vi "A3-GPS-Decoder.vi"(2 "ASCII Hexidecimal String":string) -> (0 "Date (YYYYMMDD)":u32, 1 "Time (HHMMSS)":u32, 3 "Longitude (Deg)":dbl, 4 "Latitude (Deg)":dbl, 5 "AMSL (m)":sgl, 6 "Velocity North (cm/s)":sgl, 7 "Velocity East (cm/s)":sgl, 8 "Velocity Down (cm/s)":sgl)   [LabVIEW 2019]
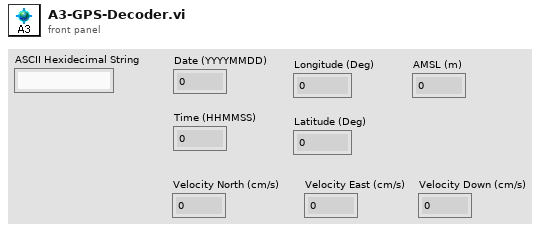
[diagram p1: front panel]
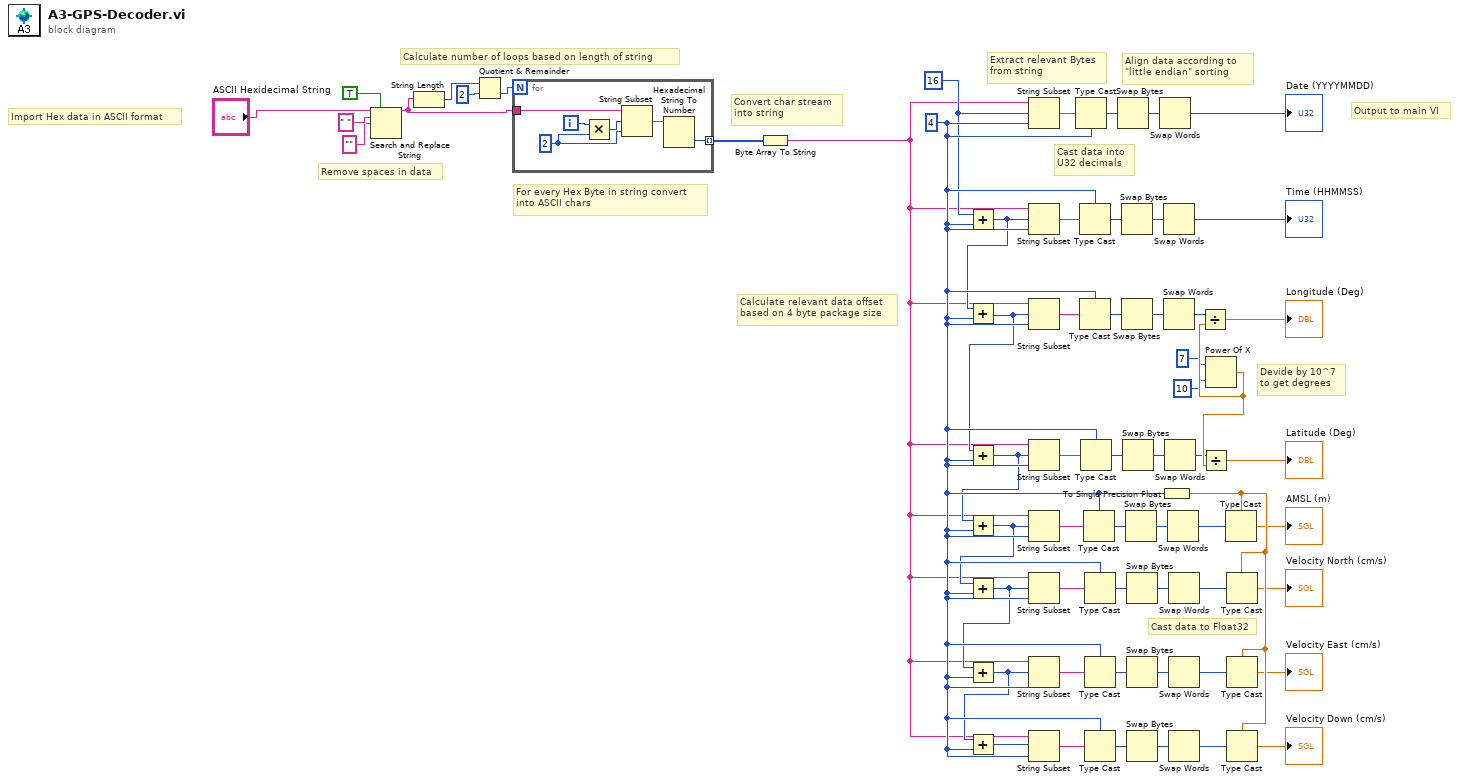
[diagram p0: block diagram]
diagram:
  w61 = u32 4 ("length (rest)")
  w20 = u32 16 ("offset (0)")
  # "Calculate relevant data offset \nbased on 4 byte package size"
  # "Cast data to Float32"
  # "Devide by 10^7 \nto get degrees"
  # "Output to main VI"
  # "Align data according to \n\"little endian\" sorting"
  # "Cast data into \nU32 decimals"
  # "Extract relevant Bytes \nfrom string"
  # "Convert char stream\ninto string"
  # "For every Hex Byte in string convert \ninto ASCII chars"
  # "Calculate number of loops based on length of string"
  # "Remove spaces in data"
  # "Import Hex data in ASCII format"
  n1 = Search and Replace String(replace all?=TRUE ("replace all? (F)"), input string="ASCII Hexidecimal String", search string=" ", replace string="" ("replace string (\"\")")) -> (result string=w3:string)  [unwired: 4 in, 3 out]
  n2 = String Length(string=w3) -> (length=w10:i32)
  n3 = Quotient & Remainder(x=w10, y=2) -> (floor(x/y)=w8:i32)  [unwired: 1 out]
  n4 = for {
    N: w8 -> [_]
    tunnel: w3 -> [w62]
    tunnel: [w63] -> w7 mode=indexing
    i -> [w66]
    w65 = 2 ("length (rest)")
    n5 = Multiply(x=w66, y=w65) -> (x*y=w67:i32)
    n6 = String Subset(string=w62, offset (0)=w67, length (rest)=w65) -> (substring=w64:string)
    n7 = Hexadecimal String To Number(string=w64) -> (number=w63:u32)  [unwired: 2 in, 1 out]
  }
  n8 = Byte Array To String(unsigned byte array=w7) -> (string=w2:string)
  n9 = Add(x=w20, y=w61) -> (x+y=w21:u32)
  n10 = Add(x=w21, y=w61) -> (x+y=w30:u32)
  n11 = Add(x=w30, y=w61) -> (x+y=w33:u32)
  n12 = Add(x=w33, y=w61) -> (x+y=w41:u32)
  n13 = Add(x=w41, y=w61) -> (x+y=w60:u32)
  n14 = Add(x=w60, y=w61) -> (x+y=w50:u32)
  n15 = Add(x=w50, y=w61) -> (x+y=w58:u32)
  n16 = String Subset(string=w2, offset (0)=w20, length (rest)=w61) -> (substring=w11:string)
  n17 = String Subset(string=w2, offset (0)=w21, length (rest)=w61) -> (substring=w51:string)
  n18 = String Subset(string=w2, offset (0)=w30, length (rest)=w61) -> (substring=w52:string)
  n19 = String Subset(string=w2, offset (0)=w33, length (rest)=w61) -> (substring=w53:string)
  n20 = String Subset(string=w2, offset (0)=w41, length (rest)=w61) -> (substring=w54:string)
  n21 = String Subset(string=w2, offset (0)=w60, length (rest)=w61) -> (substring=w55:string)
  n22 = String Subset(string=w2, offset (0)=w50, length (rest)=w61) -> (substring=w56:string)
  n23 = String Subset(string=w2, offset (0)=w58, length (rest)=w61) -> (substring=w57:string)
  n24 = Type Cast(type=w61, x=w11) -> (*(type *) &x=w13:u32)
  n25 = Type Cast(type=w61, x=w51) -> (*(type *) &x=w16:u32)
  n26 = Type Cast(type=w61, x=w52) -> (*(type *) &x=w19:u32)
  n27 = Type Cast(type=w61, x=w53) -> (*(type *) &x=w27:u32)
  n28 = Type Cast(type=w61, x=w54) -> (*(type *) &x=w34:u32)
  n29 = Type Cast(type=w61, x=w55) -> (*(type *) &x=w38:u32)
  n30 = Type Cast(type=w61, x=w56) -> (*(type *) &x=w43:u32)
  n31 = Type Cast(type=w61, x=w57) -> (*(type *) &x=w47:u32)
  n32 = Swap Bytes(anything=w13) -> (byte swapped=w12:u32)
  n33 = Swap Bytes(anything=w16) -> (byte swapped=w15:u32)
  n34 = Swap Bytes(anything=w19) -> (byte swapped=w18:u32)
  n35 = Swap Bytes(anything=w27) -> (byte swapped=w26:u32)
  n36 = Swap Bytes(anything=w34) -> (byte swapped=w32:u32)
  n37 = Swap Bytes(anything=w38) -> (byte swapped=w37:u32)
  n38 = Swap Bytes(anything=w43) -> (byte swapped=w42:u32)
  n39 = Swap Bytes(anything=w47) -> (byte swapped=w46:u32)
  n40 = Swap Words(1:w12) -> (0:→"Date (YYYYMMDD)":u32)
  n41 = To Single Precision Float(number=w61) -> (single precision float=w59:sgl)
  n42 = Swap Words(1:w15) -> (0:→"Time (HHMMSS)":u32)
  n43 = Swap Words(1:w18) -> (0:w24:u32)
  n44 = Swap Words(1:w26) -> (0:w28:u32)
  n45 = Swap Words(1:w32) -> (0:w36:u32)
  n46 = Swap Words(1:w37) -> (0:w40:u32)
  n47 = Swap Words(1:w42) -> (0:w45:u32)
  n48 = Swap Words(1:w46) -> (0:w49:u32)
  n49 = Power Of X(1:10 ("x"), 2:7 ("y")) -> (0:w31:dbl)
  n50 = Divide(x=w24, y=w31) -> (x/y=→"Longitude (Deg)":dbl)
  n51 = Divide(x=w28, y=w31) -> (x/y=→"Latitude (Deg)":dbl)
  n52 = Type Cast(type=w59, x=w36) -> (*(type *) &x=→"AMSL (m)":sgl)
  n53 = Type Cast(type=w59, x=w40) -> (*(type *) &x=→"Velocity North (cm/s)":sgl)
  n54 = Type Cast(type=w59, x=w45) -> (*(type *) &x=→"Velocity East (cm/s)":sgl)
  n55 = Type Cast(type=w59, x=w49) -> (*(type *) &x=→"Velocity Down (cm/s)":sgl)
